vi "Get Session Info.vi"   [LabVIEW 2020, in "MeasurementLink Session Management.lvlib" / "Session Reservation.lvclass"]
doc: "Gets the session information for the session reservation."
uses:
  Session Reservation.lvclass
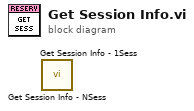
[diagram p0: block diagram]
diagram:
  n1 = call "Get Session Info - NSess .vi"() -> ()  [unwired: 9 in, 3 out]
  n2 = call "Get Session Info - 1Sess .vi"() -> ()  [unwired: 9 in, 3 out]
